vi "Sub_Pin_Location_to_Node2.vi"(10 "Pin Location":dbl, 11 "Setup Parameters":T1) -> (3 "DOF of Interest":i32)   [LabVIEW 2021]
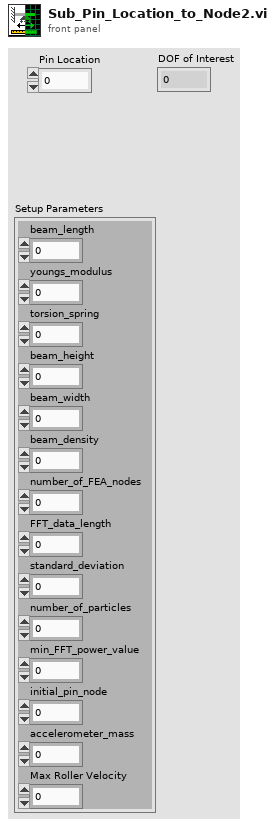
[diagram p1: front panel]
types:
  T1 = cluster{"beam_length":dbl, "youngs_modulus":dbl, "torsion_spring":dbl, "beam_height":dbl, "beam_width":dbl, "beam_density":dbl, "number_of_FEA_nodes":i32, "FFT_data_length":i32, "standard_deviation":dbl, "number_of_particles":i32, "min_FFT_power_value":dbl, "initial_pin_node":i32, "accelerometer_mass":dbl, "Max Roller Velocity":dbl}
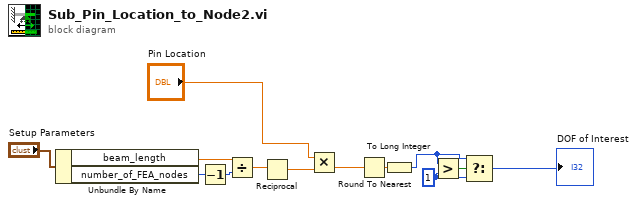
[diagram p0: block diagram]
diagram:
  w9 = 1 ("y")
  n1 = Unbundle By Name("Setup Parameters") -> ("beam_length"=w5:dbl, "number_of_FEA_nodes"=w7:i32)
  n2 = Decrement(x=w7) -> (x-1=w6:i32)
  n3 = Divide(x=w5, y=w6) -> (x/y=w2:dbl)
  n4 = Reciprocal(x=w2) -> (1/x=w1:dbl)
  n5 = Multiply(x="Pin Location", y=w1) -> (x*y=w4:dbl)
  n6 = Round To Nearest(number=w4) -> (nearest integer value=w13:dbl)
  n7 = To Long Integer(number=w13) -> (32bit integer=w11:i32)
  n8 = Greater?(x=w11, y=w9) -> (0:w12:bool)
  n9 = Select(t=w11, s=w12, f=w9) -> (s? t:f=→"DOF of Interest":i32)
